vi "FTW-Container-Object-ToContainer.vi"(0 "Names":string[](array[string]), 5 "Values":variant[](array[variant]), 11 "error in":errorcluster) -> (4 "?":variant, 15 "error out":errorcluster)   [LabVIEW 2015, in "FTW-Container.lvclass"]
uses:
  FTW-Container.lvclass
  FTW-Container-Object.ctl
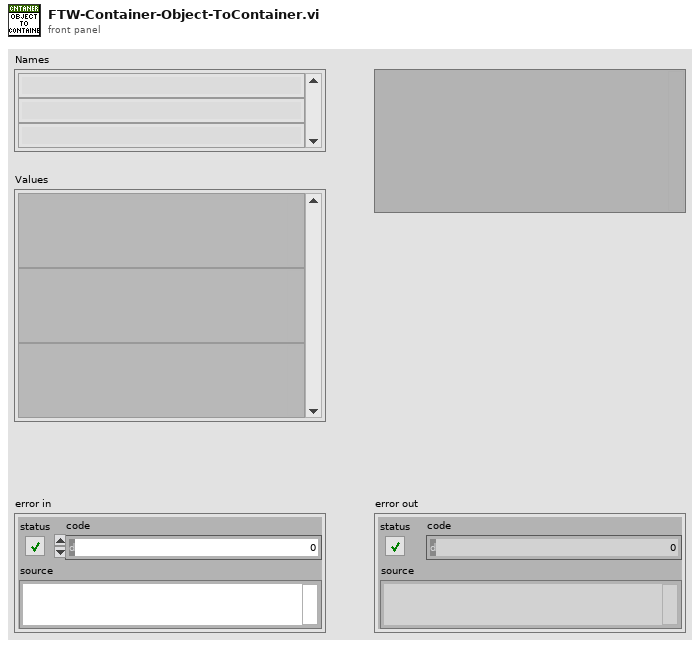
[diagram p1: front panel]
types:
  T1 = typedef "FTW-Container.lvclass/FTW-Container-Object.ctl" = cluster{"Names":string[], "Values":variant[]}
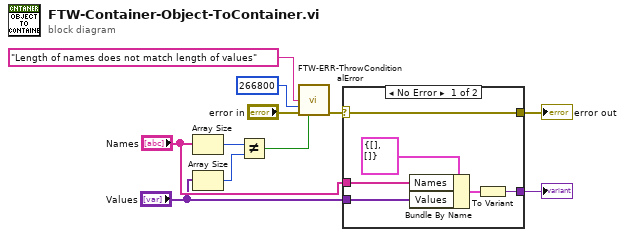
[diagram p0: block diagram]
diagram:
  n1 = Array Size(array="Names") -> (size(s)=w6:i32)
  n2 = Array Size(array="Values") -> (size(s)=w5:i32)
  n3 = Not Equal?(x=w6, y=w5) -> (x != y?=w4:bool)
  n4 = call "FTW-ERR-ThrowConditionalError.vi"("Error Message"="Length of names does not match length of values", "Error Code"=266800, "error in"="error in", "Throw Error?"=w4) -> ("error out"=w7:errorcluster)  [unwired: 11 in]
  n5 = case shown="No Error" w7 {
    selector: w7 -> [w12 w18]
    tunnel: [w15 _] -> w11
    tunnel: "Names" -> [w14 _]
    tunnel: "Values" -> [w13 _]
    tunnel: [w12 w18] -> w1
    frame No Error {
      n6 = Bundle By Name(cluster=T1 {"Names"=[], "Values"=[]}, "Names"=w14, "Values"=w13) -> (w16:T1)
      n7 = To Variant(anything=w16) -> (Variant=w15:variant)
    }
    frame Error {
    }
  }
  "error out" <- w1
  "?" <- w11
